vi "Final Project.vi"() -> ()   [LabVIEW 2019]
uses:
  <vilib>/sound2/lvsound2.llb/Sound Data Format.ctl
  <vilib>/sound2/lvsound2.llb/Sampling Mode.ctl
  <vilib>/measure/maspectr.llb/FFT Power Spectrum and PSD for 1 Chan.vi
  <vilib>/sound2/lvsound2.llb/Sound File Write Open.vi
  <vilib>/sound2/lvsound2.llb/Sound File Write (DBL).vi
  <vilib>/sound2/lvsound2.llb/Sound Input Read (DBL).vi
  <vilib>/express/express analysis/Spectral/Block/exnSpectralBlock spectral measurements peak poly.vi
  <vilib>/express/express analysis/Spectral/Block/exnSpectralBlock spectral measurements peak DDT.vi
  <vilib>/express/express analysis/Spectral/XNode/ExpressSpectralMeasurementsBlockNode.xnode
  <vilib>/measure/NI_MAPro.lvlib
panel:
  out "FTT (Peak)":dynamicdata(graph)
  out "Error":bool
  out "Waveform Graph":waveform(dbl)[](graph)
  out "Error":bool
  in  "stop":bool
  in  "number of samples/ch":i32=100000
  in  "device ID":u32
  in  "sound format":T1={"sample rate (S/s)"=22050.0, "number of channels"=2, "bits per sample"=16}
  out "Time Stamp":dynamicdata(graph)
  in  "Discard Transient":i32 caption="Begin Sample"
  out "x*y":dbl
  out "Recorded Input":dynamicdata(graph)
  out "max index(es)":i32
  out "magnitude of each frequency":dbl[](array[numeric])
  out "FTT Spectrum":cluster{"f0":dbl, "df":dbl, "magnitude":dbl[]}(graph)
  # "maximum value excluding the DC\noffset that is occuring in the signal"
  # "The max amplitude of the\nincoming frequencies"
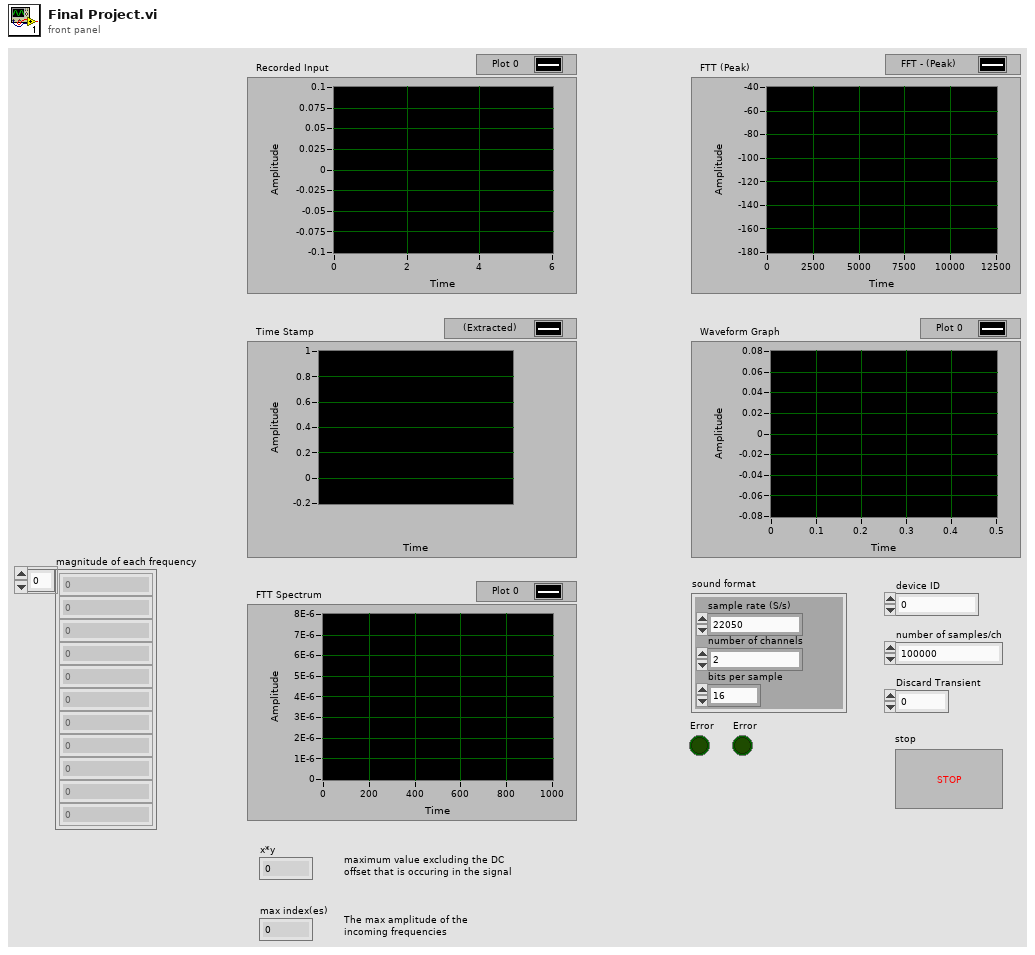
[diagram p1: front panel]
types:
  T1 = typedef "Sound Data Format.ctl" = cluster{"sample rate (S/s)":dbl, "number of channels":i32, "bits per sample":i32}
  T2 = typedef "Sampling Mode.ctl" = i32
  T3 = typedef "Sound File Refnum.ctl" = refnum<file>
  T4 = typedef "Sound Input Task ID.ctl" = u32
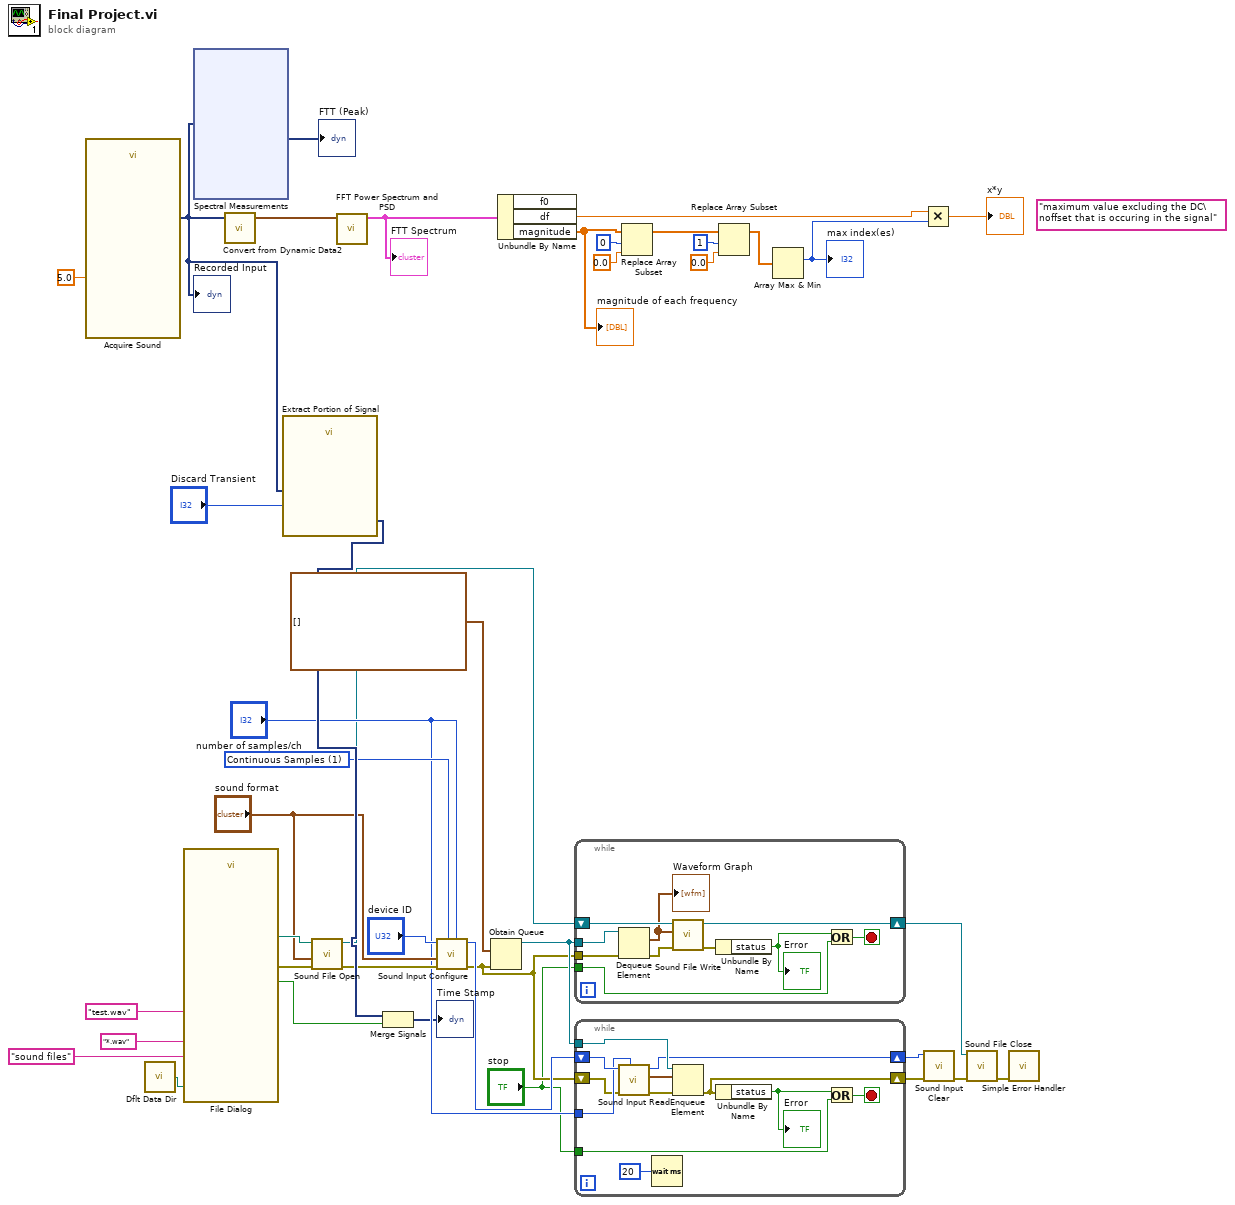
[diagram p0: block diagram]
diagram:
  (unwired) "maximum value excluding the DC\noffset that is occuring in the signal"
  w20 = T2 1 items=["Finite Samples", "Continuous Samples"] ("sample mode")
  n1 = call "Acquire Sound"("Duration (s)"=5.0) -> ("Data"=w3:dynamicdata)  [unwired: 17 in, 1 out]
  "Recorded Input" <- w3
  n2 = call <vilib>:"Dflt Data Dir.vi"() -> ("App:Default Data Directory"=w26:path)
  n3 = call "File Dialog"("start path"=w26, "default name"="test.wav", "pattern (all files)"="*.wav", "pattern label"="sound files") -> ("selected path"=w22:path, "exists"=w15:bool, "error out"=w21:errorcluster)  [unwired: 8 in, 1 out]
  n4 = xnode "Spectral Measurements"("Signals"=w3) -> ("FFT - (Peak)"=→"FTT (Peak)":dynamicdata)  [unwired: 1 in, 2 out]
  n5 = call "Convert from Dynamic Data2"("Dynamic Data Type"=w3) -> ("Waveform"=w40:waveform(dbl))  [unwired: 3 in]
  n6 = call "Extract Portion of Signal"("Begin Sample"="Discard Transient", "Signals"=w3) -> ("Section"=w27:dynamicdata)  [unwired: 8 in, 1 out]
  n7 = call-poly <vilib>:"Sound File Open.vi"("error in (no error)"=w21, "sound format"="sound format", "path"=w22) -> ("error out"=w17:errorcluster, "sound file refnum"=w8:T3)  [unwired: 7 in]
  n8 = call-poly <vilib>:"FFT Power Spectrum and PSD.vi"("time signal"=w40) -> ("Power Spectrum / PSD"=w41:cluster{"f0":dbl, "df":dbl, "magnitude":dbl[]})  [unwired: 7 in, 3 out]
  "FTT Spectrum" <- w41
  n9 = Merge Signals(w27, w15) -> (→"Time Stamp":dynamicdata)
  n10 = call <vilib>:"Sound Input Configure.vi"("number of samples/ch"="number of samples/ch", "sample mode"=w20, "error in (no error)"=w17, "sound format"="sound format", "device ID"="device ID") -> ("error out"=w6:errorcluster, "task ID"=w14:T4)  [unwired: 5 in]
  n11 = Obtain Queue(element data type=waveform(dbl)[] [] ("data"), error in (no error)=w6) -> (queue out=w7:refnum<queue>)  [unwired: 3 in, 2 out]
  n12 = Unbundle By Name(w41) -> ("df"=w31:dbl, "magnitude"=w39:dbl[])  [unwired: 1 out]
  "magnitude of each frequency" <- w39
  n13 = while {
    shift-right: [w44] -> w5
    shift-left: w8 -> [w48]
    tunnel: w7 -> [w51]
    tunnel: w6 -> [w50]
    tunnel: "stop" -> [w42]
    stop <- w46 stop-if-true
    n14 = Dequeue Element(queue=w51, error in (no error)=w50) -> (element=w47:waveform(dbl)[], error out=w49:errorcluster)  [unwired: 1 in, 2 out]
    "Waveform Graph" <- w47
    n15 = call-poly <vilib>:"Sound File Write.vi"("error in (no error)"=w49, "data"=w47, "sound file refnum"=w48) -> ("error out"=w43:errorcluster, "sound file refnum out"=w44:T3)  [unwired: 7 in]
    n16 = Unbundle By Name(w43) -> ("status"=w45:bool)
    "Error" <- w45
    n17 = Or(x=w45, y=w42) -> (x .or. y?=w46:bool)
  }
  n18 = while {
    shift-right: [w57] -> w12
    shift-left: w14 -> [w63]
    shift-right: [w56] -> w11
    shift-left: w6 -> [w61]
    tunnel: "number of samples/ch" -> [w62]
    tunnel: w7 -> [w58]
    tunnel: "stop" -> [w52]
    stop <- w55 stop-if-true
    n19 = call-poly <vilib>:"Sound Input Read.vi"("number of samples/ch"=w62, "error in (no error)"=w61, "task ID"=w63) -> ("error out"=w60:errorcluster, "data"=w59:waveform(dbl)[], "task ID out"=w57:T4)  [unwired: 6 in]
    n20 = Wait (ms)(milliseconds to wait=u32 20) -> ()  [unwired: 1 out]
    n21 = Enqueue Element(queue=w58, element=w59, error in (no error)=w60) -> (error out=w56:errorcluster)  [unwired: 1 in, 2 out]
    n22 = Unbundle By Name(w56) -> ("status"=w54:bool)
    "Error" <- w54
    n23 = Or(x=w54, y=w52) -> (x .or. y?=w55:bool)
  }
  n24 = Replace Array Subset(array=w39, new element=0.0 ("new element/subarray"), index=0) -> (w36:dbl[])
  n25 = Replace Array Subset(array=w36, new element=0.0 ("new element/subarray"), index=1) -> (w33:dbl[])
  n26 = Array Max & Min(array=w33) -> (max index (indices)=w32:i32)  [unwired: 3 out]
  "max index(es)" <- w32
  n27 = Multiply(x=w31, y=w32) -> (x*y=→"x*y":dbl)
  n28 = call <vilib>:"Sound Input Clear.vi"("error in (no error)"=w11, "task ID"=w12) -> ("error out"=w10:errorcluster)  [unwired: 9 in]
  n29 = call <vilib>:"Sound File Close.vi"("error in (no error)"=w10, "sound file refnum"=w5) -> ("error out"=w9:errorcluster)  [unwired: 9 in]
  n30 = call <vilib>:"Simple Error Handler.vi"("error in (no error)"=w9) -> ()  [unwired: 4 in, 5 out]
